vi "QueryNames.vi"(8 "error in (no error)":errorcluster, 10 "TableName(\"\")":string, 11 "ExcuseNotes in":refnum<class "ExcuseNotesHandler.lvclass">) -> (0 "error out":errorcluster, 2 "Names(\"\")":string[](array[string]), 3 "ExcuseNotes out":refnum<class "ExcuseNotesHandler.lvclass">)   [LabVIEW 2015, in "ExcuseNotesHandler.lvclass"]
uses:
  ExcuseNotesHandler.lvclass
  ExcuseNotesHandler.lvclass/ExcuseNotesHandler.ctl
  API/_Database/Database.lvclass
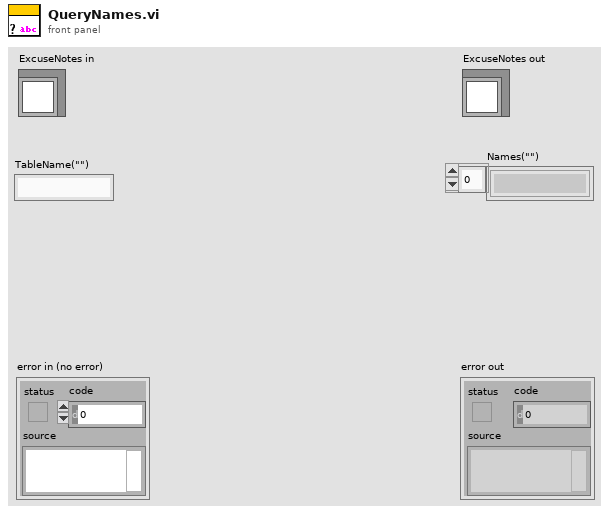
[diagram p1: front panel]
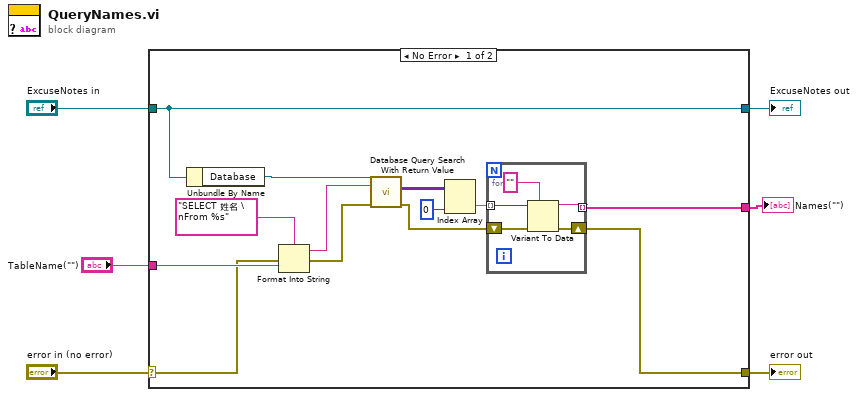
[diagram p0: block diagram]
diagram:
  n1 = case shown="No Error" "error in (no error)" {
    selector: "error in (no error)" -> [w14 w26]
    tunnel: [w8 w26] -> w5
    tunnel: [w19 w25] -> w3
    tunnel: "ExcuseNotes in" -> [w19 w25]
    tunnel: "TableName(\"\")" -> [w15 _]
    tunnel: [w7 _] -> w1
    frame No Error {
      n2 = Unbundle By Name(w19) -> ("Database"=w18:refnum<class "Database.lvclass">)
      n3 = Format Into String(format string="SELECT 姓名 \nFrom %s" ("SQL query"), error in=w14, w15) -> (resulting string=w16:string, error out=w13:errorcluster)  [unwired: 1 in]
      n4 = call "Database Query Search With Return Value.vi"("error in (no error)"=w13, "SQL query"=w16, "object in"=w18) -> ("error out"=w9:errorcluster, "recordset data"=w12:variant[][])  [unwired: 5 in, 2 out]
      n5 = Index Array(array=w12, index (col)=0 ("disabled index (col)")) -> (element=w10:variant[])  [unwired: 1 in]
      n6 = for {
        tunnel: w10 -> [w24] mode=indexing
        shift-right: [w21] -> w8
        shift-left: w9 -> [w22]
        tunnel: [w20] -> w7 mode=indexing
        n7 = Variant To Data(error in=w22, type="", Variant=w24) -> (data=w20:string, error out=w21:errorcluster)
      }
    }
    frame Error {
    }
  }
  "error out" <- w5
  "ExcuseNotes out" <- w3
  "Names(\"\")" <- w1
